vi "Form Initial Report String.vi"(11 "Library Name":string) -> (3 "String":string)   [LabVIEW 2019]
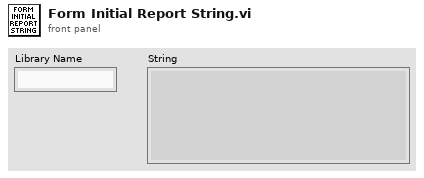
[diagram p1: front panel]
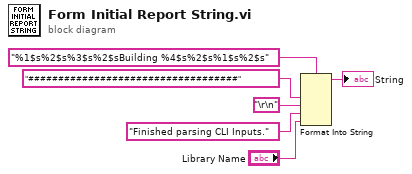
[diagram p0: block diagram]
diagram:
  n1 = Format Into String(format string="%1$s%2$s%3$s%2$sBuilding %4$s%2$s%1$s%2$s", "###################################", "\r\n", "Finished parsing CLI Inputs." ("Text to Write"), "Library Name") -> (resulting string=→"String":string)  [unwired: 2 in, 1 out]
